vi "MyTopic ComplexType Reader Example.vi"() -> ()   [LabVIEW 2016]
uses:
  subVIs/MyTopic ComplexType.ctl
  <vilib>/RTI DDS Toolkit/Types/RTI DDS Advanced Reader Configuration.ctl
  <vilib>/RTI DDS Toolkit/Library/LVDDS_library.lvlib
panel:
  out "error out":errorcluster
  in  "Advanced Reader Configuration":T1
  in  "Domain Id":u32
  in  "Topic Name":string="MyTopicWriter"
  out "complexType":T2={"I32_Num"=0, "I64_Num"=0, "U16_Num"=0, "Sgl_Array"=[1.0, 1.0, 1.0, 1.0], "innercluster"={"Sgl_Num"=0.0, "Boolean"=FALSE}}
  in  "MyComplexType type":T2={"I32_Num"=0, "I64_Num"=0, "U16_Num"=0, "Sgl_Array"=[1.0, 1.0, 1.0, 1.0], "innercluster"={"Sgl_Num"=0.0, "Boolean"=FALSE}}
  in  "error in (no error)":errorcluster
  in  "Stop Reading":bool
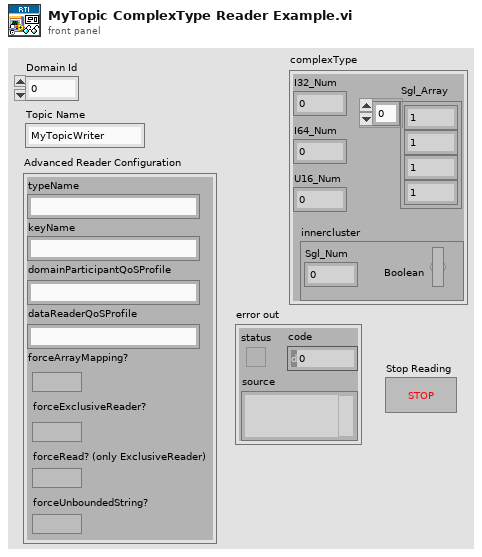
[diagram p1: front panel]
types:
  T1 = typedef "LVDDS_library.lvlib/RTI DDS Advanced Reader Configuration.ctl" = cluster{"typeName":string, "keyName":string, "domainParticipantQoSProfile":string, "dataReaderQoSProfile":string, "forceArrayMapping?":bool, "forceExclusiveReader?":bool, "forceRead? (only ExclusiveReader)":bool, "forceUnboundedString?":bool}
  T2 = typedef "MyTopic ComplexType.ctl" = cluster{"I32_Num":i32, "I64_Num":i64, "U16_Num":u16, "Sgl_Array":sgl[], "innercluster":cluster{"Sgl_Num":sgl, "Boolean":bool}}
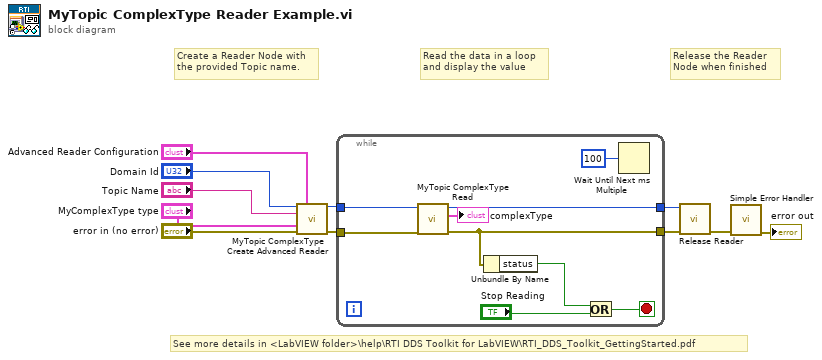
[diagram p0: block diagram]
diagram:
  # "See more details in <LabVIEW folder>\\help\\RTI DDS Toolkit for LabVIEW\\RTI_DDS_Toolkit_GettingStarted.pdf"
  # "Release the Reader \nNode when finished"
  # "Read the data in a loop \nand display the value"
  # "Create a Reader Node with\nthe provided Topic name."
  n1 = call "MyTopic ComplexType Create Advanced Reader.vi"("Domain Id"="Domain Id", "Advanced Reader Configuration"="Advanced Reader Configuration", "Topic Name"="Topic Name", "MyComplexType type"="MyComplexType type", "error in (no error)"="error in (no error)") -> ("Refnum"=w8:u64, "error out"=w7:errorcluster)  [unwired: 9 in]
  n2 = while "Main Loop" {
    tunnel: w8 -> [w20]
    tunnel: [w18] -> w11
    tunnel: w7 -> [w17]
    tunnel: [w13] -> w10
    stop <- w14 stop-if-true
    n3 = call "MyTopic ComplexType Read.vi"("error in"=w17, "DDS Object Ref"=w20) -> ("error out"=w13:errorcluster, "complexType"=→"complexType":T2, "DDS Object Ref out"=w18:u64)  [unwired: 6 in, 1 out]
    n4 = Unbundle By Name(w13) -> ("status"=w16:bool)
    n5 = Or(x=w16, y="Stop Reading") -> (x .or. y?=w14:bool)
    n6 = Wait Until Next ms Multiple(millisecond multiple=u32 100) -> ()  [unwired: 1 out]
  }
  n7 = call <vilib>:"Release Reader.vi"("error in (no error)"=w10, "DDS Object Ref"=w11) -> ("error out"=w9:errorcluster)  [unwired: 9 in]
  n8 = call <vilib>:"Simple Error Handler.vi"("error in (no error)"=w9) -> ("error out"=→"error out":errorcluster)  [unwired: 4 in, 4 out]
